vi "Process.vi"(8 "error in":errorcluster, 11 "Logger.Error":refnum<class "Logger.Error.lvclass">) -> (0 "error out":errorcluster, 3 "Logger.Error out":refnum<class "Logger.Error.lvclass">)   [LabVIEW 2019, in "Logger.Error.lvclass"]
doc: "---------------------------------------------------------------\nJKI State Machine Objects™\nhttp://jki.net/state-machine-objects/\nCopyright (C) 2005-2015, JKI <info@jki.net>\nALL RIGHTS RESERVED"
uses:
  Logger.Error.lvclass
  C:/Program Files (x86)/National Instruments/LabVIEW 2019/vi.lib/JKI/JKI SMO/SMO/SMO.lvclass
  C:/Users/patrick/Documents/GitHub/Instrument-Framework/lvsrc/SMOs/Logger/Logger.lvclass
  <vilib>/JKI/JKI SMO/SMO/Typedefs/Parent Call--Enum.ctl
  <vilib>/JKI/JKI SMO/SMO/SMO.lvclass/SMO.ctl
  Logger.Error.lvclass/Logger.Error.ctl
  <vilib>/JKI/JKI SMO/SMO/Private/ReftoDVR--SMO.vi
  Logger/Logger.lvclass
  <vilib>/JKI/JKI SMO/SMO/SMO.lvclass
  <userlib>/_MGI/Error Reporter/MGI Error Reporter Base/MGI Error Reporter Base.lvclass
panel:
  # "For instructions on how to use the JKI State Machine Objects, examples and video tutorials, visit:\nhttp://jki.net/state-machine-objects/\n\nJKI State Machine Objects™\nhttp://jki.net/state-machine-objects/\nCopyright (C) 2005-2015, JKI <info@jki.net>\nALL RIGHTS RESERVED"
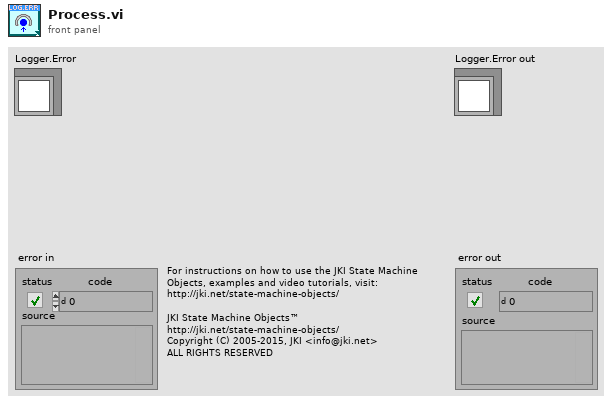
[diagram p1: front panel]
types:
  T1 = typedef "SMO.lvclass/Parent Call--Enum.ctl" = enum16{"Allows parent to run", "Does not request parent to run"}
  T2 = enum32{"invalid app kind", "Development System", "Run Time System", "Student Edition", "Embedded LabVIEW", "Evaluation", "Custom"}
  T3 = enum32{"Invalid", "Standard", "Closed", "Hidden", "Minimized", "Maximized"}
  T4 = enum32{"Bad", "Idle", "Run top level", "Running"}
  T5 = cluster{"Core":cluster{"Current VI Reference":refnum<vi>, "Close Panel on Exit?":bool, "error":errorcluster}, "Self Reference":refnum<class "Logger.Error.lvclass">, "path":path, "Debug Mode?":bool}
  T6 = cluster{"Current VI Reference":refnum<vi>, "Close Panel on Exit?":bool, "error":errorcluster}
  T7 = typedef "SMO.lvclass/Protected Events.ctl" = cluster{"StopProcesses":refnum<user-event>, "AbortProcesses":refnum<user-event>, "Config Changed":refnum<user-event>, "Dependency":refnum<user-event>}
  T8 = typedef "SMO.lvclass/Public Events.ctl" = cluster{"Error":refnum<user-event>, "State":refnum<user-event>, "Reserve State":refnum<user-event>}
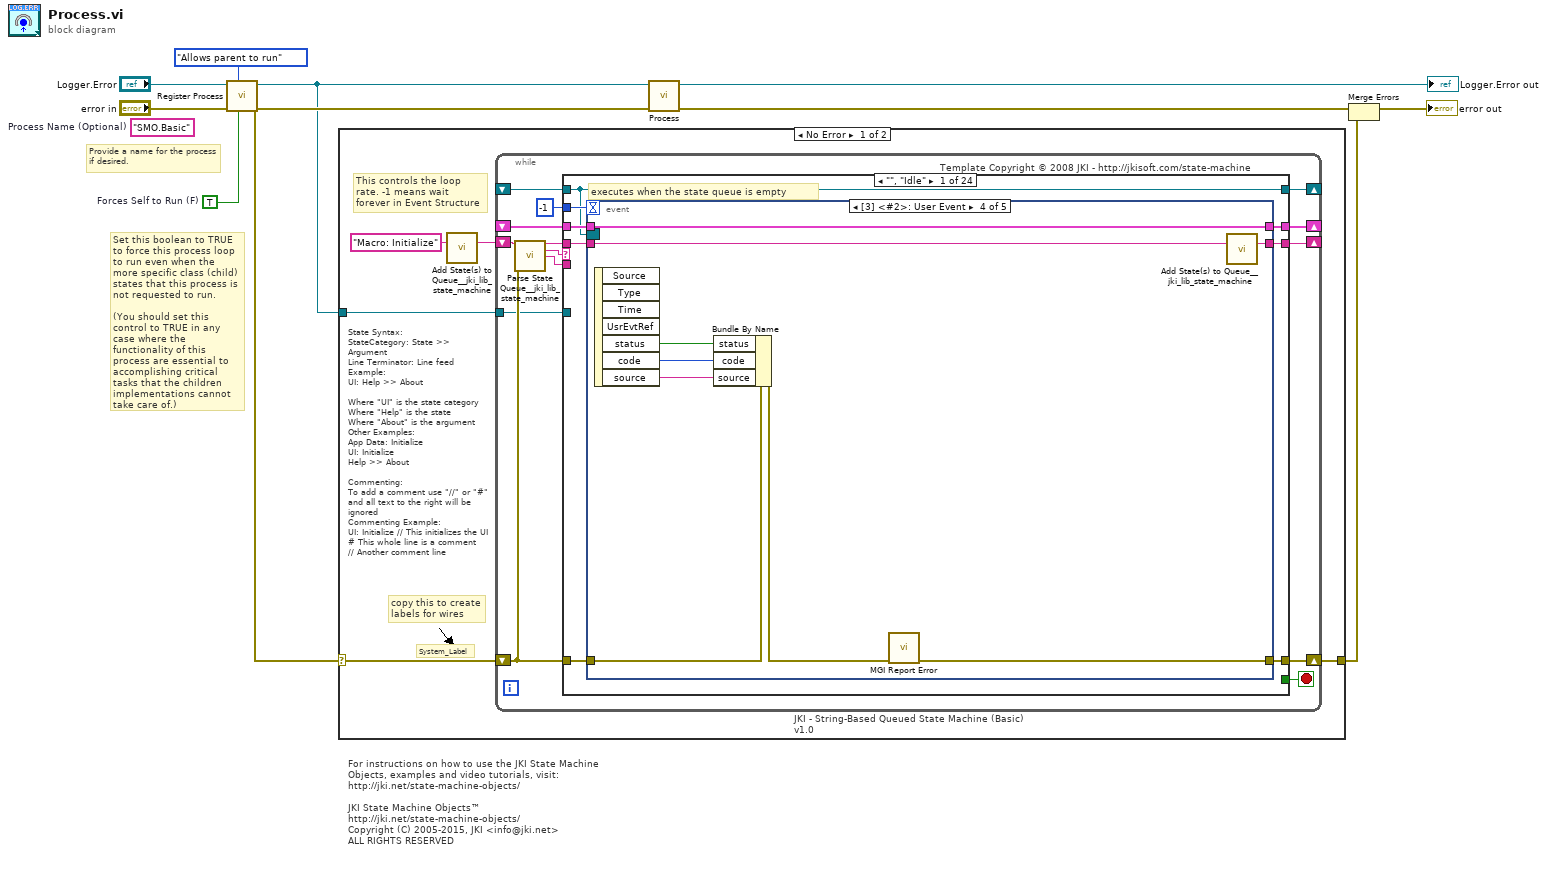
[diagram p0: block diagram]
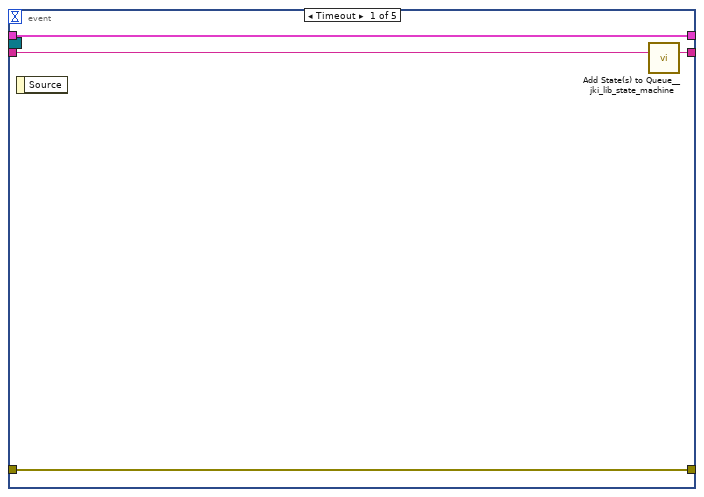
[diagram p2: hidden frame]
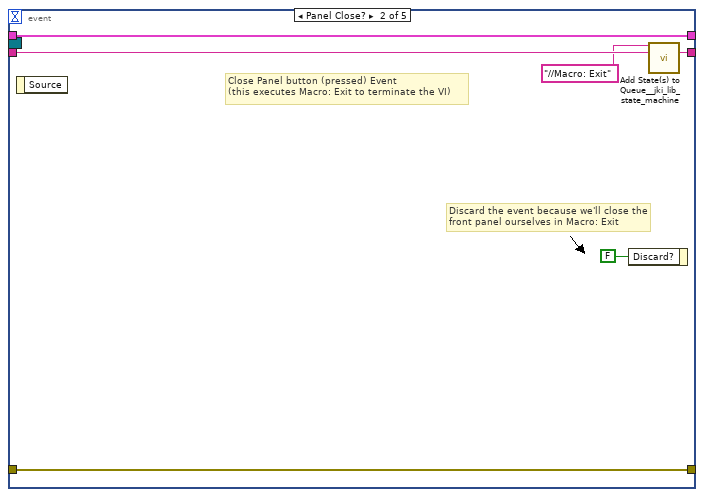
[diagram p3: hidden frame]
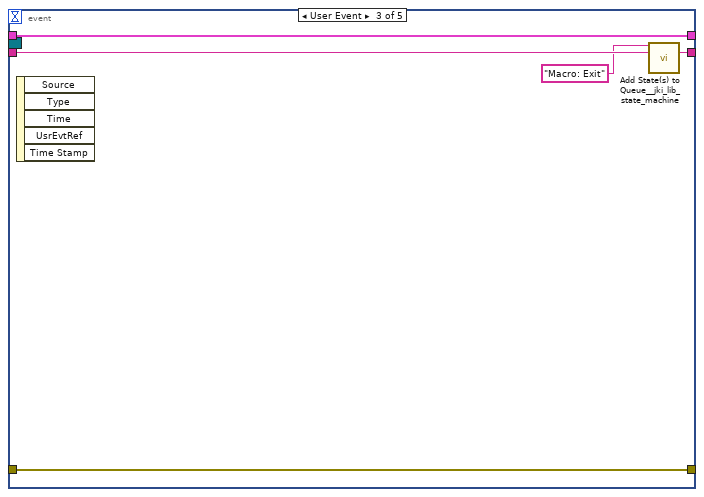
[diagram p4: hidden frame]
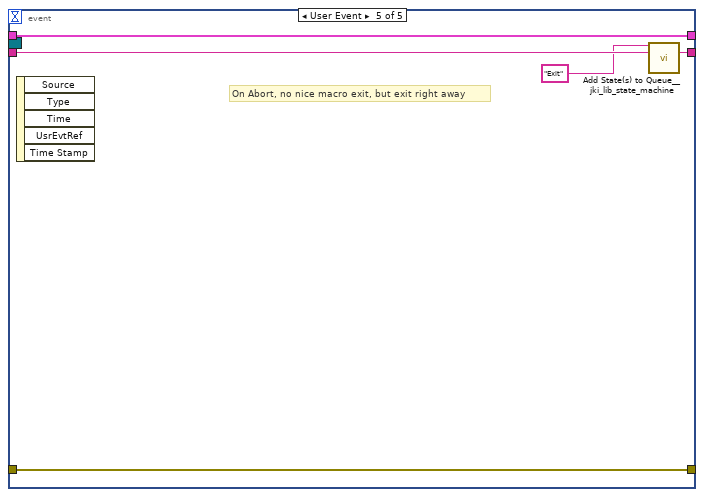
[diagram p5: hidden frame]
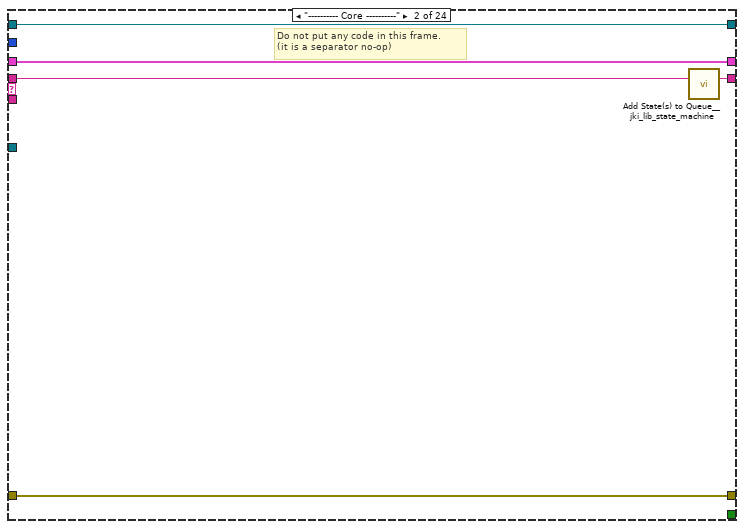
[diagram p6: hidden frame]
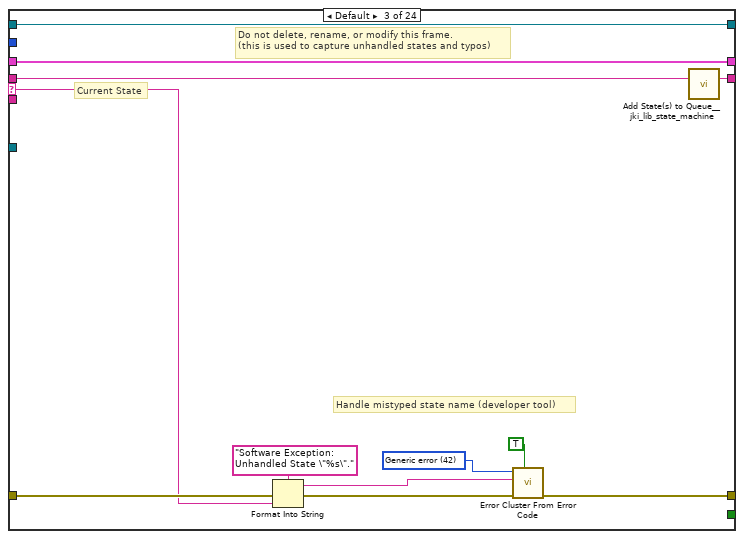
[diagram p7: hidden frame]
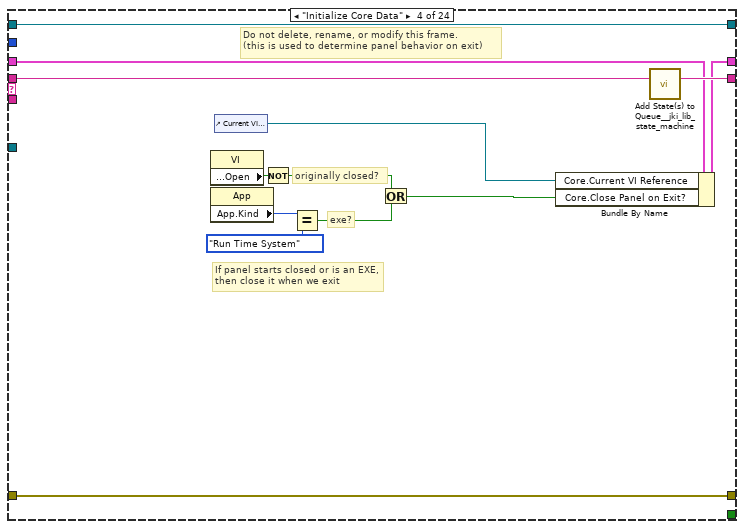
[diagram p8: hidden frame]
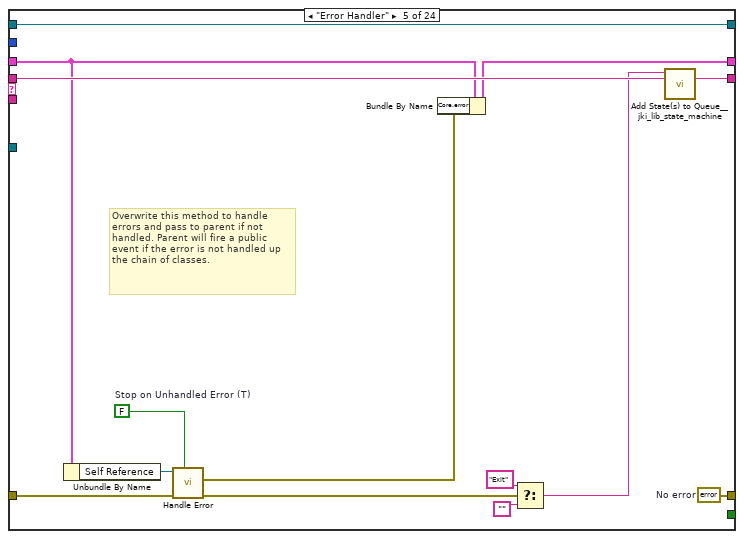
[diagram p9: hidden frame]
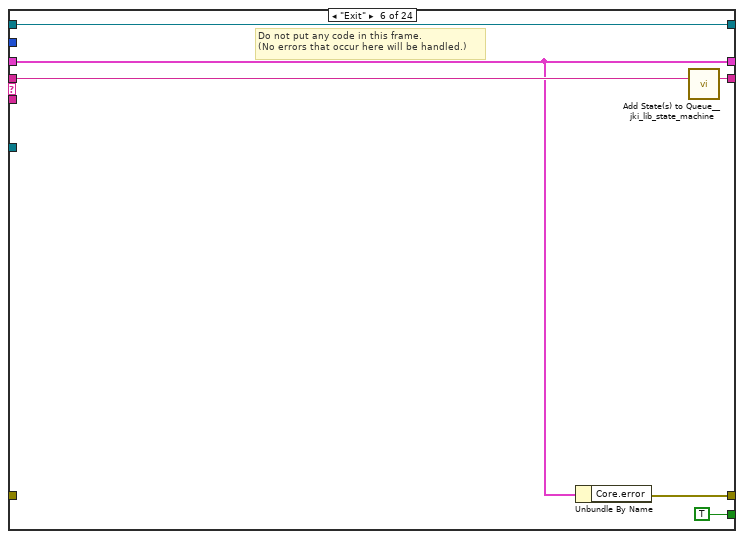
[diagram p10: hidden frame]
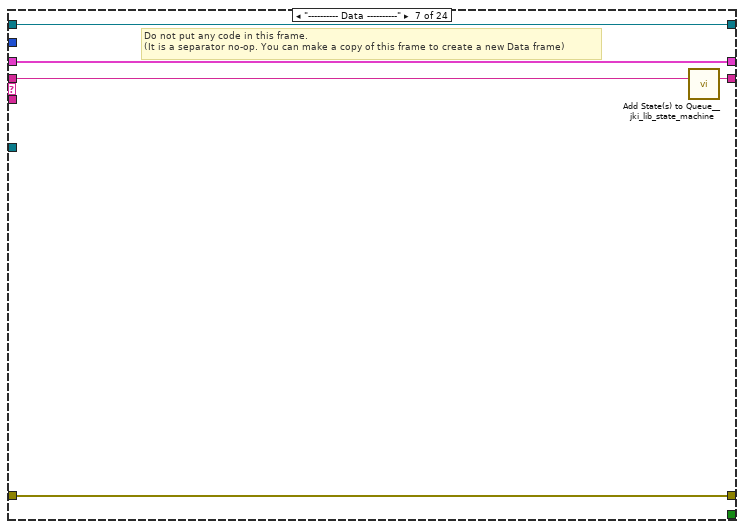
[diagram p11: hidden frame]
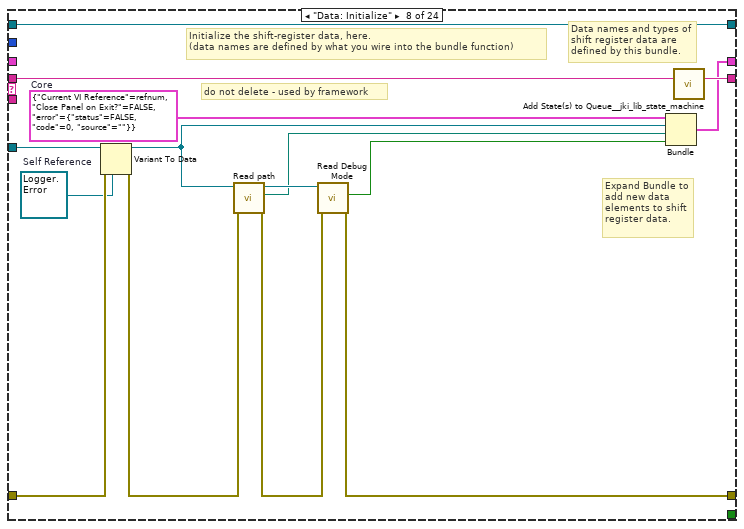
[diagram p12: hidden frame]
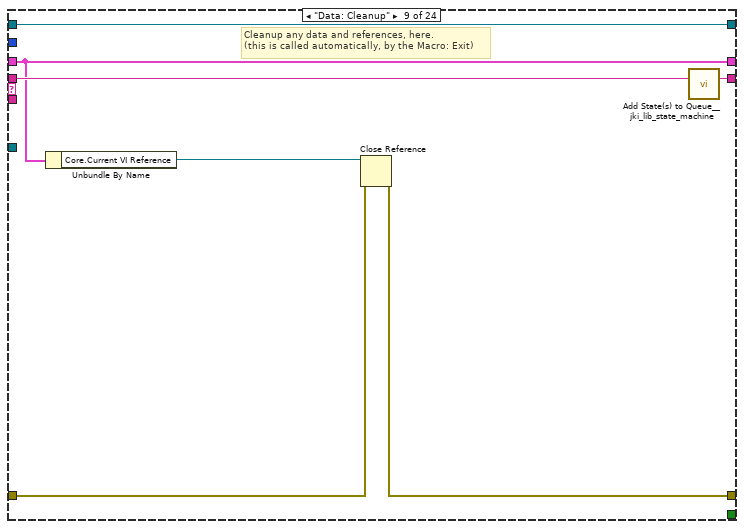
[diagram p13: hidden frame]
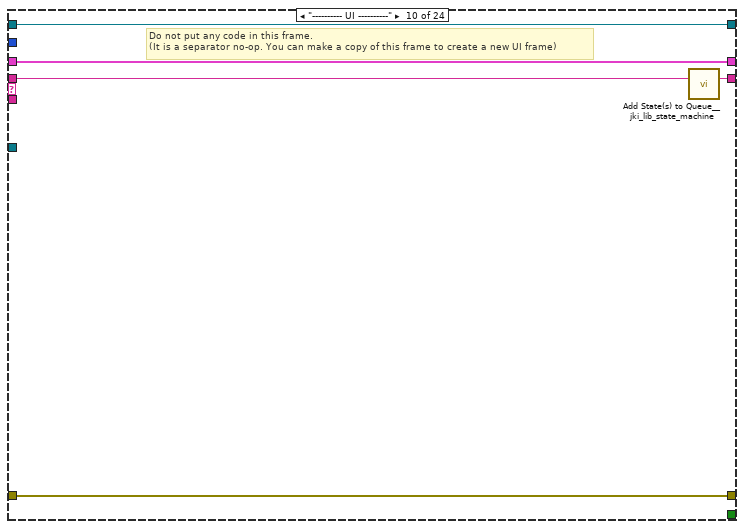
[diagram p14: hidden frame]
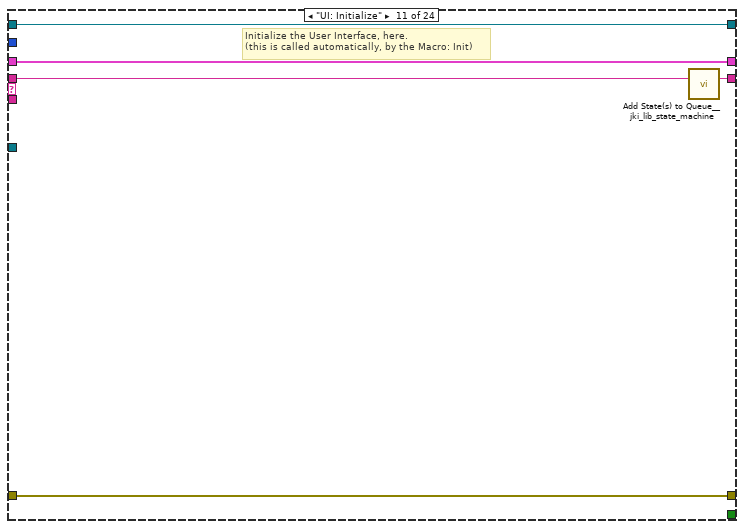
[diagram p15: hidden frame]
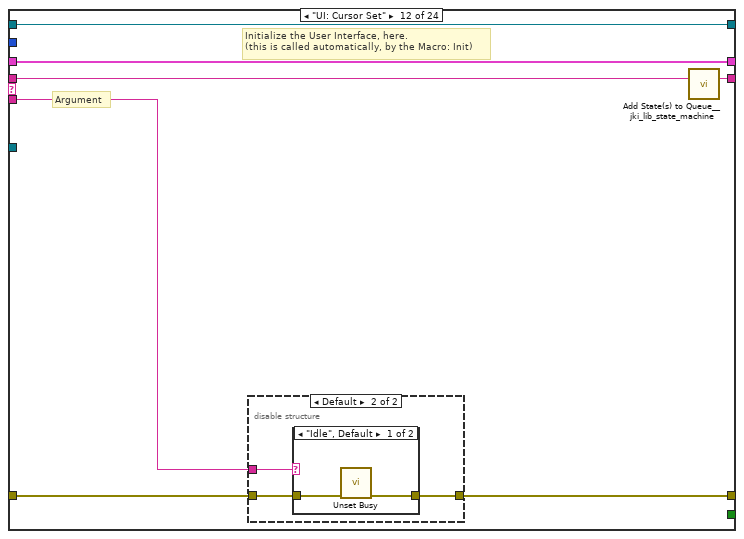
[diagram p16: hidden frame]
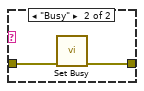
[diagram p18: hidden frame]
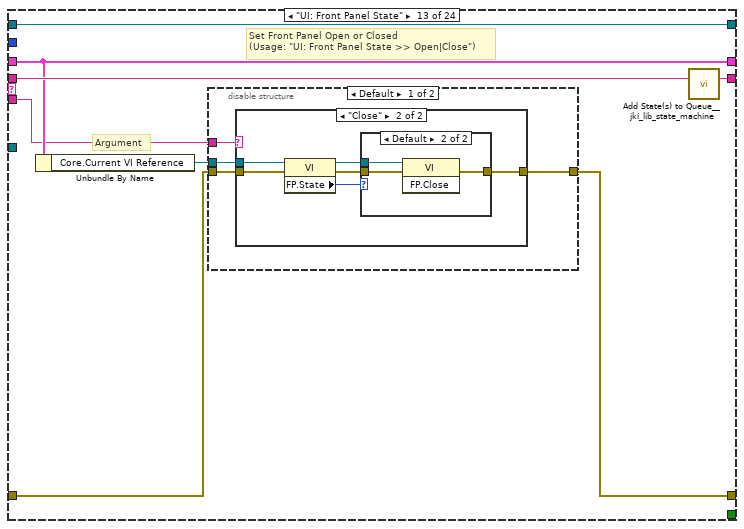
[diagram p19: hidden frame]
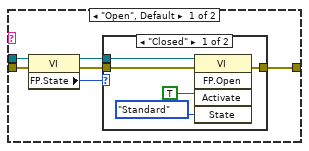
[diagram p20: hidden frame]
diagram:
  w1 = TRUE  # Forces Self to Run (F)
  (unwired) "SMO.Basic"  # Process Name (Optional)
  # "Provide a name for the process\nif desired."
  # "Set this boolean to TRUE to force this process loop to run even when the more specific class (child) states that this process is not requested to run.\n\n(You should set this control to TRUE in any case where the functionality of this process are essential to accomplishing critical tasks that the children implementations cannot take care of.)"
  # "For instructions on how to use the JKI State Machine Objects, examples and video tutorials, visit:\nhttp://jki.net/state-machine-objects/\n\nJKI State Machine Objects™\nhttp://jki.net/state-machine-objects/\nCopyright (C) 2005-2015, JKI <info@jki.net>\nALL RIGHTS RESERVED"
  n1 = call <vilib>:"Register Process.vi"("Forces Self to Run (F)"=w1, "Parent Call"=Parent_Call--Enum."Allows parent to run", "error in (no error)"="error in", "SMO"="Logger.Error") -> ("error out"=w7:errorcluster, "SMO out"=w6:refnum<class "Logger.Error.lvclass">)  [unwired: 6 in]
  n2 = case shown="No Error" w7 {
    selector: w7 -> [w12 w320]
    tunnel: w6 -> [w13 _]
    tunnel: [w11 w320] -> w3
    frame No Error {
      # "State Syntax:\nStateCategory: State >> Argument\nLine Terminator: Line feed\nExample:\nUI: Help >> About\n\nWhere \"UI\" is the state category\nWhere \"Help\" is the state\nWhere \"About\" is the argument\nOther Examples:\nApp Data: Initialize\nUI: Initialize\nHelp >> About\n\nCommenting:\nTo add a comment use \"//\" or \"#\" and all text to the right will be ignored\nCommenting Example:\nUI: Initialize // This initializes the UI\n# This whole line is a comment\n// Another comment line"
      # "copy this to create labels for wires"
      # "This controls the loop rate. -1 means wait forever in Event Structure"
      # "System_Label"
      n3 = call <vilib>:"Add State(s) to Queue__jki_lib_state_machine.vi"("State(s) in (\"\")"="Macro: Initialize") -> ("States Out"=w15:string)  [unwired: 14 in]
      n4 = while "JKI - String-Based Queued State Machine (Basic) v1.0" {
        shift-right: [w22] -> _
        shift-left: _ -> [w21]
        shift-right: [w25] -> w11
        shift-left: w12 -> [w19]
        shift-right: [w24] -> _
        shift-left: w15 -> [w26]
        tunnel: w13 -> [w18]
        shift-right: [w17] -> _
        shift-left: _ -> [w16]
        stop <- w23 stop-if-true
        # "Template Copyright © 2008 JKI - http://jkisoft.com/state-machine"
        n5 = call <vilib>:"Parse State Queue__jki_lib_state_machine.vi"("State Queue"=w26, "Error In (no error)"=w19) -> ("Remaining States"=w28:string, "Current State"=w29:string, "Arguments"=w27:string)  [unwired: 11 in]
        n6 = case shown="\"\", \"Idle\"" w29 {
          selector: w29 -> [_ _ w73 _ _ _ _ _ _ _ _ _ _ _ _ _ _ _ _ _ _ _ _ _]
          tunnel: w28 -> [w37 w71 w77 w96 w110 w116 w121 w136 w143 w148 w153 w160 w176 w208 w231 w251 w256 w267 w272 w290 w300 w305 w312 w319]
          tunnel: w27 -> [_ _ _ _ _ _ _ _ _ _ _ w154 w170 _ _ _ _ _ _ _ _ _ _ _]
          tunnel: w21 -> [w35 w68 w75 w87 w104 w112 w118 _ w138 w145 w151 w158 w172 w205 w214 w243 w253 w264 w269 w288 w298 w303 w309 w316]
          tunnel: [w34 w69 w79 w93 w105 w111 w119 w122 w139 w146 w150 w155 w173 w206 w211 w249 w254 w258 w270 w284 w296 w301 w307 w313] -> w25
          tunnel: w19 -> [w33 w69 w78 w93 w106 _ w119 w133 w140 w146 w150 w156 w174 w206 w210 w249 w254 w259 w270 w285 w296 w301 w308 w314]
          tunnel: [w36 w70 w76 w95 w109 w115 w120 w135 w142 w147 w152 w159 w175 w207 w230 w250 w255 w266 w271 w289 w299 w304 w311 w318] -> w24
          tunnel: [_ _ _ _ _ TRUE _ _ _ _ _ _ _ _ _ _ _ _ _ _ _ _ _ _] -> w23
          tunnel: [w32 w68 w75 w94 w103 w112 w118 w134 w138 w145 w151 w158 w172 w205 w214 w243 w253 w264 w269 w288 w298 w303 w309 w316] -> w22
          tunnel: -1 ("Timeout") -> [w31 _ _ _ _ _ _ _ _ _ _ _ _ _ _ _ _ _ _ _ _ _ _ _]
          tunnel: w18 -> [_ _ _ _ _ _ _ w131 _ _ _ _ _ _ w212 _ _ _ _ _ _ _ _ _]
          tunnel: [w30 w67 w72 w84 w108 w113 w117 w130 w137 w144 w149 w157 w169 w204 w229 w244 w252 w265 w268 w287 w297 w302 w310 w317] -> w17
          tunnel: w16 -> [w30 w67 w72 w84 w108 w113 w117 w130 w137 w144 w149 w157 w169 w204 w229 w244 w252 w265 w268 _ w297 w302 w310 w317]
          frame "", "Idle" {
            # "executes when the state queue is empty"
            n7 = event shown="[3] <#2>: User Event" {
              selector: w30 -> [_ _ _ _ _]
              dyn-events: _ -> [_ _ _ _ _]
              timeout: w31 -> [_ _ _ _ _]
              tunnel: w37 -> [w41 w47 w52 w61 w66]
              tunnel: [w40 w46 w51 w60 w65] -> w36
              tunnel: w35 -> [w39 w44 w49 w59 w63]
              tunnel: [w38 w45 w50 w53 w64] -> w34
              tunnel: w33 -> [w38 w45 w50 w55 w64]
              tunnel: [w39 w44 w49 w59 w63] -> w32
              event Timeout {
                n8 = event-data() -> ()  [unwired: 1 in, 1 out]
                n9 = call <vilib>:"Add State(s) to Queue__jki_lib_state_machine.vi"("State(s) in (\"\")"=w41) -> ("States Out"=w40:string)  [unwired: 14 in]
              }
              event Panel Close? {
                # "Discard the event because we'll close the front panel ourselves in Macro: Exit"
                # "Close Panel button (pressed) Event\n(this executes Macro: Exit to terminate the VI)"
                n10 = event-data() -> ()  [unwired: 1 in, 1 out]
                n11 = event-data("Discard?"=FALSE) -> ()  [unwired: 1 in, 1 out]
                n12 = call <vilib>:"Add State(s) to Queue__jki_lib_state_machine.vi"("State(s) in Front (\"\")"="//Macro: Exit", "State(s) in (\"\")"=w47) -> ("States Out"=w46:string)  [unwired: 13 in]
              }
              event User Event {
                n13 = event-data() -> ()  [unwired: 1 in, 5 out]
                n14 = call <vilib>:"Add State(s) to Queue__jki_lib_state_machine.vi"("State(s) in Front (\"\")"="Macro: Exit", "State(s) in (\"\")"=w52) -> ("States Out"=w51:string)  [unwired: 13 in]
              }
              event User Event {
                n15 = event-data() -> ("status"=w58:bool, "code"=w57:i32, "source"=w56:string)  [unwired: 1 in, 4 out]
                n16 = Bundle By Name(cluster=w55, "status"=w58, "code"=w57, "source"=w56) -> (w54:errorcluster)
                n17 = call <userlib>:"MGI Report Error.vi"("error in"=w54) -> ("no error"=w53:errorcluster)  [unwired: 10 in]
                n18 = call <vilib>:"Add State(s) to Queue__jki_lib_state_machine.vi"("State(s) in (\"\")"=w61) -> ("States Out"=w60:string)  [unwired: 14 in]
              }
              event User Event {
                # "On Abort, no nice macro exit, but exit right away"
                n19 = event-data() -> ()  [unwired: 1 in, 5 out]
                n20 = call <vilib>:"Add State(s) to Queue__jki_lib_state_machine.vi"("State(s) in Front (\"\")"="Exit", "State(s) in (\"\")"=w66) -> ("States Out"=w65:string)  [unwired: 13 in]
              }
            }
          }
          frame "---------- Core ----------" {
            # "Do not put any code in this frame.\n(it is a separator no-op)"
            n21 = call <vilib>:"Add State(s) to Queue__jki_lib_state_machine.vi"("State(s) in (\"\")"=w71) -> ("States Out"=w70:string)  [unwired: 14 in]
          }
          frame Default {
            w82 = 42 items=["No error", "Argument error", "Memory is full", "Out of zone", "End of file", "File already open", "Generic file I/O error", "File not found", "File permission error", "Disk is full", "Duplicate path", "Too many files open", "System feature not enabled", "Resource file not found", "Cannot add resource", "Resource not found", "Image not found", "Image memory error", "Pen does not exist", "Config type invalid", "Config token not found", "Config parse error", "Config memory error", "Bad external code format", "Bad external code offset", "External code not present", "Null window", "Destroy window error", "Null menu", "Print aborted", "Bad print record", "Print driver error", "Windows error during printing", "Memory error during printing", "Print dialog error", "Generic print error", "Invalid device refnum", "Device not found", "Device parameter error", "Device unit error", "Cannot open device", "Device call aborted", "Generic error", "Cancelled by user", "Object ID too low", "Object ID too high", "Object not in heap", "Unknown heap", "Unknown object (invalid DefProc)", "Unknown object (DefProc not in table)", "Message out of range", "Invalid (null) method", "Unknown message", "Manager call not supported", "Bad address", "Network operation in progress", "Network operation timed out", "Connection is busy", "Network attribute not supported", "Network error", "Address in use", "System out of memory", "Connection aborted", "Connection refused", "Not connected", "Already connected", "Connection closed", "Initialization error (interapplication manager)", "Bad occurrence", "Wait on unbound occurrence handler", "Occurrence queue overflow", "Datalog type conflict", "Unused", "Unrecognized type (interapplication manager)", "Memory corrupt", "Failed to make temporary DLL", "Old CIN version", "Drag socket not found", "Failed to load drop-object", "Failed to register OLE object", "Failed to release OLE object", "Format specifier type mismatch", "Unknown format specifier", "Too few format specifiers", "Too many format specifiers", "Scan failed", "Newer CIN version", "Error converting to variant", "Runtime menu error", "Password tampered", "Variant attribute not found", "Incompatible variant data type", "Event data is not available", "Event Store is not present", "Occurrence is not found", "Event Queue is not created", "Event info is not available", "Refnum passed is NULL", "Error retrieving Class GUID", "Error retrieving CoClass GUID", "Error retrieving TypeLib GUID.", "Bad built application magic bytes.", "Specific driver is different from the specific driver associated with the Logical Name.", "There is no session opened to the class driver.", "Max Error", "MAX - Error with config objects", "MAX - Error loading configuration", "MAX - Group not supported"]
            # "Current State"
            # "Do not delete, rename, or modify this frame.\n(this is used to capture unhandled states and typos)"
            # "Handle mistyped state name (developer tool)"
            n22 = Format Into String(format string="Software Exception: Unhandled State \"%s\"." ("message"), error in=w78, w73) -> (resulting string=w81:string, error out=w80:errorcluster)  [unwired: 1 in]
            n23 = call <vilib>:"Error Cluster From Error Code.vi"("show call chain? (False)"=TRUE, "error in (no error)"=w80, "error message (\"\")"=w81, "error code (0)"=w82) -> ("error out"=w79:errorcluster)  [unwired: 5 in]
            n24 = call <vilib>:"Add State(s) to Queue__jki_lib_state_machine.vi"("State(s) in (\"\")"=w77) -> ("States Out"=w76:string)  [unwired: 14 in]
          }
          frame "Initialize Core Data" {
            # "Do not delete, rename, or modify this frame.\n(this is used to determine panel behavior on exit)"
            # "originally closed?"
            # "exe?"
            # "If panel starts closed or is an EXE, then close it when we exit"
            n25 = property class="VI"() -> ("Front Panel.Open"=w92:bool)  [unwired: 2 in, 2 out]
            n26 = property class="App"() -> ("App.Kind"=w91:T2)  [unwired: 2 in, 2 out]
            n27 = control-ref of="Current VI Reference"() -> (w85:refnum<vi>)
            n28 = Not(x=w92) -> (.not. x?=w89:bool)
            n29 = Equal?(x=w91, y=T2."Run Time System" ("Application:Kind")) -> (x = y?=w88:bool)
            n30 = Or(x=w89, y=w88) -> (x .or. y?=w86:bool)
            n31 = Bundle By Name(cluster=w87, "Core.Current VI Reference"=w85, "Core.Close Panel on Exit?"=w86) -> (w94:T5)
            n32 = call <vilib>:"Add State(s) to Queue__jki_lib_state_machine.vi"("State(s) in (\"\")"=w96) -> ("States Out"=w95:string)  [unwired: 14 in]
          }
          frame "Error Handler" {
            w97 = FALSE  # Stop on Unhandled Error (T)
            w105 = errorcluster {"status"=FALSE, "code"=0, "source"=""}  # No error
            # "Overwrite this method to handle errors and pass to parent if not handled. Parent will fire a public event if the error is not handled up the chain of classes."
            n33 = Unbundle By Name(w104) -> ("Self Reference"=w107:refnum<class "Logger.Error.lvclass">)
            n34 = call-dynamic "Handle Error.vi"("Stop on Unhandled Error (T)"=w97, "error in"=w106, "SMO"=w107) -> ("handling error"=w98:errorcluster, "Unhandled error"=w101:errorcluster)  [unwired: 6 in, 1 out]
            n35 = Bundle By Name(cluster=w104, "Core.error"=w101) -> (w103:T5)
            n36 = Select(t="Exit", s=w98, f="") -> (s? t:f=w102:string)
            n37 = call <vilib>:"Add State(s) to Queue__jki_lib_state_machine.vi"("State(s) in Front (\"\")"=w102, "State(s) in (\"\")"=w110) -> ("States Out"=w109:string)  [unwired: 13 in]
          }
          frame "Exit" {
            # "Do not put any code in this frame.\n(No errors that occur here will be handled.)"
            n38 = Unbundle By Name(w112) -> ("Core.error"=w111:errorcluster)
            n39 = call <vilib>:"Add State(s) to Queue__jki_lib_state_machine.vi"("State(s) in (\"\")"=w116) -> ("States Out"=w115:string)  [unwired: 14 in]
          }
          frame "---------- Data ----------" {
            # "Do not put any code in this frame.\n(It is a separator no-op. You can make a copy of this frame to create a new Data frame)"
            n40 = call <vilib>:"Add State(s) to Queue__jki_lib_state_machine.vi"("State(s) in (\"\")"=w121) -> ("States Out"=w120:string)  [unwired: 14 in]
          }
          frame "Data: Initialize" {
            w129 = T6 {"Current VI Reference"=refnum, "Close Panel on Exit?"=FALSE, "error"={"status"=FALSE, "code"=0, "source"=""}}  # Core
            w132 = refnum<class "Logger.Error.lvclass"> refnum  # Self Reference
            # "do not delete - used by framework"
            # "Expand Bundle to add new data elements to shift register data."
            # "Data names and types of shift register data are defined by this bundle."
            # "Initialize the shift-register data, here.\n(data names are defined by what you wire into the bundle function)"
            n41 = Variant To Data(error in=w133, type=w132, Variant=w131) -> (data=w128:refnum<class "Logger.Error.lvclass">, error out=w127:errorcluster)
            n42 = call-dynamic "Read path.vi"("error in (no error)"=w127, "Logger in"=w128) -> ("error out"=w124:errorcluster, "path"=w123:path, "Logger out"=w126:refnum<class "Logger.Error.lvclass">)  [unwired: 7 in]
            n43 = call "Read Debug Mode.vi"("error in (no error)"=w124, "Logger in"=w126) -> ("error out"=w122:errorcluster, "Debug Mode?"=w125:bool)  [unwired: 7 in, 1 out]
            n44 = Bundle("Core"=w129, "Self Reference"=w128, "path"=w123, "Debug Mode?"=w125) -> (w134:T5)  [unwired: 1 in]
            n45 = call <vilib>:"Add State(s) to Queue__jki_lib_state_machine.vi"("State(s) in (\"\")"=w136) -> ("States Out"=w135:string)  [unwired: 14 in]
          }
          frame "Data: Cleanup" {
            # "Cleanup any data and references, here.\n(this is called automatically, by the Macro: Exit)"
            n46 = Unbundle By Name(w138) -> ("Core.Current VI Reference"=w141:refnum<vi>)
            n47 = Close Reference(reference=w141, error in (no error)=w140) -> (error out=w139:errorcluster)
            n48 = call <vilib>:"Add State(s) to Queue__jki_lib_state_machine.vi"("State(s) in (\"\")"=w143) -> ("States Out"=w142:string)  [unwired: 14 in]
          }
          frame "---------- UI ----------" {
            # "Do not put any code in this frame.\n(It is a separator no-op. You can make a copy of this frame to create a new UI frame)"
            n49 = call <vilib>:"Add State(s) to Queue__jki_lib_state_machine.vi"("State(s) in (\"\")"=w148) -> ("States Out"=w147:string)  [unwired: 14 in]
          }
          frame "UI: Initialize" {
            # "Initialize the User Interface, here.\n(this is called automatically, by the Macro: Init)"
            n50 = call <vilib>:"Add State(s) to Queue__jki_lib_state_machine.vi"("State(s) in (\"\")"=w153) -> ("States Out"=w152:string)  [unwired: 14 in]
          }
          frame "UI: Cursor Set" {
            # "Argument"
            # "Initialize the User Interface, here.\n(this is called automatically, by the Macro: Init)"
            n51 = disable-structure shown="Default" {
              disable-tunnel: w156 -> [w161 w164]
              disable-tunnel: [w161 w163] -> w155
              disable-tunnel: w154 -> [_ w162]
              frame condition #0 {
              }
              frame condition #1 (active) {
                n52 = case shown="\"Idle\", Default" w162 {
                  tunnel: w164 -> [w166 w168]
                  tunnel: [w165 w167] -> w163
                  frame "Idle", Default {
                    n53 = call <vilib>:"Unset Busy.vi"("error in (no error)"=w166) -> ("error out"=w165:errorcluster)  [unwired: 10 in]
                  }
                  frame "Busy" {
                    n54 = call <vilib>:"Set Busy.vi"("error in (no error)"=w168) -> ("error out"=w167:errorcluster)  [unwired: 9 in, 1 out]
                  }
                }
              }
            }
            n55 = call <vilib>:"Add State(s) to Queue__jki_lib_state_machine.vi"("State(s) in (\"\")"=w160) -> ("States Out"=w159:string)  [unwired: 14 in]
          }
          frame "UI: Front Panel State" {
            # "Argument"
            # "Set Front Panel Open or Closed\n(Usage: \"UI: Front Panel State >> Open|Close\")"
            n56 = Unbundle By Name(w172) -> ("Core.Current VI Reference"=w171:refnum<vi>)
            n57 = disable-structure shown="Default" {
              disable-tunnel: w174 -> [w180 w203]
              disable-tunnel: [w179 w203] -> w173
              disable-tunnel: w171 -> [w178 _]
              disable-tunnel: w170 -> [w177 _]
              frame condition #0 (active) {
                n58 = case shown="\"Close\"" w177 {
                  tunnel: w180 -> [w184 w197]
                  tunnel: [w186 w198] -> w179
                  tunnel: w178 -> [w185 w195]
                  frame "Open", Default {
                    n59 = property class="VI"(reference=w185, error in=w184) -> (reference out=w182:refnum<vi>, error out=w183:errorcluster, "FP.State"=w181:T3)
                    n60 = case shown="\"Closed\"" w181 {
                      tunnel: [w189 w192] -> w186
                      tunnel: w183 -> [w188 w192]
                      tunnel: w182 -> [w187 _]
                      frame "Closed" {
                        n61 = invoke class="VI" method="FP.Open"(reference=w187, error in=w188, "Activate"=TRUE, "State"=T3."Standard") -> (error out=w189:errorcluster)  [unwired: 1 in, 4 out]
                      }
                      frame Default {
                      }
                    }
                  }
                  frame "Close" {
                    n62 = property class="VI"(reference=w195, error in=w197) -> (reference out=w194:refnum<vi>, error out=w196:errorcluster, "FP.State"=w193:T3)
                    n63 = case shown="Default" w193 {
                      tunnel: [w199 w202] -> w198
                      tunnel: w196 -> [w199 w201]
                      tunnel: w194 -> [_ w200]
                      frame "Invalid", "Closed" {
                      }
                      frame Default {
                        n64 = invoke class="VI" method="FP.Close"(reference=w200, error in=w201) -> (error out=w202:errorcluster)  [unwired: 1 in, 2 out]
                      }
                    }
                  }
                }
              }
              frame condition #1 {
              }
            }
            n65 = call <vilib>:"Add State(s) to Queue__jki_lib_state_machine.vi"("State(s) in (\"\")"=w176) -> ("States Out"=w175:string)  [unwired: 14 in]
          }
          frame "---------- Macro ----------" {
            # "Do not put any code in this frame.\n(It is a separator no-op. You can make a copy of this frame to create a new Macro frame)"
            n66 = call <vilib>:"Add State(s) to Queue__jki_lib_state_machine.vi"("State(s) in (\"\")"=w208) -> ("States Out"=w207:string)  [unwired: 14 in]
          }
          frame "Macro: Initialize" {
            w221 = "Process: Sync"
            # "This needs to be called here before Data: Initialize\nto ensure that the correct argument is present"
            # "Initialization Macro\n(This is called once, when the VI starts)"
            n67 = control-ref of="This VI"() -> (w223:refnum<vi>)
            n68 = property class="VI"(reference=w223) -> ("Exec.State"=w222:T4)  [unwired: 1 in, 2 out]
            n69 = call "Read Debug Mode.vi"("error in (no error)"=w210, "Logger in"=w212) -> ("error out"=w211:errorcluster, "Debug Mode?"=w209:bool)  [unwired: 7 in, 1 out]
            n70 = Equal?(x=w222, y=T4."Run top level") -> (x = y?=w227:bool)
            n71 = Select(t="Open", s=w209, f="Close") -> (s? t:f=w218:string)
            n72 = call <vilib>:"Build State String with Arguments__JKI_lib_State_Machine.vi"("Arguments (\"\")"=w218, "State"="UI: Front Panel State") -> ("State with Arguments"=w215:string)  [unwired: 4 in]
            n73 = Select(t=w221, s=w227, f="") -> ()  [unwired: 1 out]
            n74 = call <vilib>:"Add State(s) to Queue__jki_lib_state_machine.vi"("State(s) in Front (\"\")"="Logger: Start Error Logger\nUI: Initialize", "State(s) in (\"\")"=w215) -> ("States Out"=w213:string)  [unwired: 13 in]
            n75 = call <vilib>:"Add State(s) to Queue__jki_lib_state_machine.vi"("State(s) in Front (\"\")"="Data: Initialize\nInitialize Core Data\nEvents: Register", "State(s) in (\"\")"=w221, "State(s) at Back (\"\")"=w213) -> ("States Out"=w224:string)  [unwired: 12 in]
            n76 = call <vilib>:"Add State(s) to Queue__jki_lib_state_machine.vi"("State(s) in Front (\"\")"=w224, "State(s) in (\"\")"=w231) -> ("States Out"=w230:string)  [unwired: 13 in]
          }
          frame "Macro: Exit" {
            # "Exit Macro\n(This is called once, when the VI exits)"
            n77 = Unbundle By Name(w243) -> ("Debug Mode?"=w232:bool, "Core.Close Panel on Exit?"=w248:bool)
            n78 = Select(t="Open", s=w232, f="Close") -> (s? t:f=w235:string)
            n79 = call <vilib>:"Build State String with Arguments__JKI_lib_State_Machine.vi"("Arguments (\"\")"=w235, "State"="UI: Front Panel State") -> ("State with Arguments"=w233:string)  [unwired: 4 in]
            n80 = Select(t=w233, s=w248, f="") -> (s? t:f=w246:string)
            n81 = call <vilib>:"Add State(s) to Queue__jki_lib_state_machine.vi"("State(s) in Front (\"\")"="Logger: Stop Error Logger\nData: Cleanup\nEvents: Unregister", "State(s) in (\"\")"="Process: Sync", "State(s) at Back (\"\")"="Exit") -> ("States Out"=w240:string)  [unwired: 12 in]
            n82 = call <vilib>:"Add State(s) to Queue__jki_lib_state_machine.vi"("State(s) in Front (\"\")"="" ("State(s) in Front (\"\")"), "State(s) in (\"\")"=w246, "State(s) at Back (\"\")"=w240) -> ("States Out"=w245:string)  [unwired: 12 in]
            n83 = call <vilib>:"Add State(s) to Queue__jki_lib_state_machine.vi"("State(s) in Front (\"\")"=w245, "State(s) in (\"\")"=w251) -> ("States Out"=w250:string)  [unwired: 13 in]
          }
          frame "---------- Process ----------" {
            # "Template Separator\n(You can make a copy of, or modify, this frame)"
            n84 = call <vilib>:"Add State(s) to Queue__jki_lib_state_machine.vi"("State(s) in (\"\")"=w256) -> ("States Out"=w255:string)  [unwired: 14 in]
          }
          frame "Process: Sync" {
            n85 = Unbundle By Name(w264) -> ("Self Reference"=w260:refnum<class "Logger.Error.lvclass">)
            n86 = call <vilib>:"WaitOnProcessSync.vi"("error in (no error)"=w259, "SMO"=w260) -> ("error out"=w258:errorcluster, "Don't run?"=w263:bool)  [unwired: 7 in, 1 out]
            n87 = Select(t="Data: Cleanup\nEvents: Unregister\nExit", s=w263, f="") -> (s? t:f=w257:string)
            n88 = call <vilib>:"Add State(s) to Queue__jki_lib_state_machine.vi"("State(s) in Front (\"\")"=w257, "State(s) in (\"\")"=w267) -> ("States Out"=w266:string)  [unwired: 13 in]
          }
          frame "---------- Events ----------" {
            # "Template Separator\n(You can make a copy of, or modify, this frame)"
            n89 = call <vilib>:"Add State(s) to Queue__jki_lib_state_machine.vi"("State(s) in (\"\")"=w272) -> ("States Out"=w271:string)  [unwired: 14 in]
          }
          frame "Events: Register" {
            # "Expand to add\nmore events"
            n90 = Unbundle By Name(w288) -> ("Self Reference"=w286:refnum<class "Logger.Error.lvclass">)
            n91 = call <vilib>:"GetProtectedEvents.vi"("SMO"=w286) -> ("error out"=w282:errorcluster, "SMO Protected Events"=w281:T7, "SMO out"=w278:refnum<class "Logger.Error.lvclass">)  [unwired: 8 in]
            n92 = Unbundle By Name(w278) -> ("SMOs"=w280:refnum<class "SMO.lvclass">[])
            n93 = for {
              tunnel: [w293] -> w275 mode=indexing
              tunnel: w280 -> [w292] mode=indexing
              tunnel: [w291] -> w279 mode=indexing
              n94 = call <vilib>:"GetPublicEvents.vi"("SMO"=w292) -> ("error out"=w291:errorcluster, "Public Events"=w294:T8)  [unwired: 8 in, 1 out]
              n95 = Unbundle By Name(w294) -> ("Error"=w293:refnum<user-event>)
            }
            n96 = call <vilib>:"GetPublicEvents.vi"("SMO"=w278) -> ("error out"=w273:errorcluster, "Public Events"=w277:T8)  [unwired: 8 in, 1 out]
            n97 = Unbundle By Name(w277) -> ("Error"=w276:refnum<user-event>)
            n98 = Build Array (concatenate)(w276, w275) -> (w274:refnum<user-event>[])
            n99 = register-events(w281, w274) -> (reference out=w287:refnum<event-registration>, error out=w283:errorcluster)  [unwired: 2 in]
            n100 = Merge Errors(w273, w279, w285, w283, w282) -> (w284:errorcluster)
            n101 = call <vilib>:"Add State(s) to Queue__jki_lib_state_machine.vi"("State(s) in (\"\")"=w290) -> ("States Out"=w289:string)  [unwired: 14 in]
          }
          frame "Events: Unregister" {
            n102 = Unregister For Events(event registration refnum=w297, error in=w296) -> (error out=w295:errorcluster)
            n103 = call <vilib>:"Clear Errors.vi"("error in (no error)"=w295) -> ()  [unwired: 5 in, 2 out]
            n104 = call <vilib>:"Add State(s) to Queue__jki_lib_state_machine.vi"("State(s) in (\"\")"=w300) -> ("States Out"=w299:string)  [unwired: 14 in]
          }
          frame "---------- Logger ----------" {
            n105 = call <vilib>:"Add State(s) to Queue__jki_lib_state_machine.vi"("State(s) in (\"\")"=w305) -> ("States Out"=w304:string)  [unwired: 14 in]
          }
          frame "Logger: Start Error Logger" {
            # "will these work with other SMOs?"
            n106 = Unbundle By Name(w309) -> ("Self Reference"=w306:refnum<class "Logger.Error.lvclass">)
            n107 = call-dynamic "Create Logger.vi"("error in (no error)"=w308, "Logger.Error in"=w306) -> ("error out"=w307:errorcluster)  [unwired: 8 in, 1 out]
            n108 = call <vilib>:"Add State(s) to Queue__jki_lib_state_machine.vi"("State(s) in (\"\")"=w312) -> ("States Out"=w311:string)  [unwired: 14 in]
          }
          frame "Logger: Stop Error Logger" {
            n109 = Unbundle By Name(w316) -> ("Self Reference"=w315:refnum<class "Logger.Error.lvclass">)
            n110 = call-dynamic "Destroy Logger.vi"("error in (no error)"=w314, "Logger.Error in"=w315) -> ("error out"=w313:errorcluster)  [unwired: 8 in, 1 out]
            n111 = call <vilib>:"Add State(s) to Queue__jki_lib_state_machine.vi"("State(s) in (\"\")"=w319) -> ("States Out"=w318:string)  [unwired: 14 in]
          }
        }
      }
    }
    frame Error {
    }
  }
  n112 = call-parent "Process.vi"("error in"=w7, "Logger"=w6) -> ("error out"=w4:errorcluster, "Logger out"=→"Logger.Error out":refnum<class "Logger.Error.lvclass">)  [unwired: 8 in]
  n113 = Merge Errors(w4, w3) -> (→"error out":errorcluster)
